vi "Main.vi"(11 "Mode":T1(ring)) -> ()   [LabVIEW 2017]
uses:
  Game Mode/Game Mode.lvclass
  Game Mode/PvP-1/Single Computer PvP.lvclass
  C:/LabVIEW Packages/Sources/GuessingGame/Game Mode/Game Mode.lvclass
panel:
  out "error out":errorcluster
  in  "Stop":bool
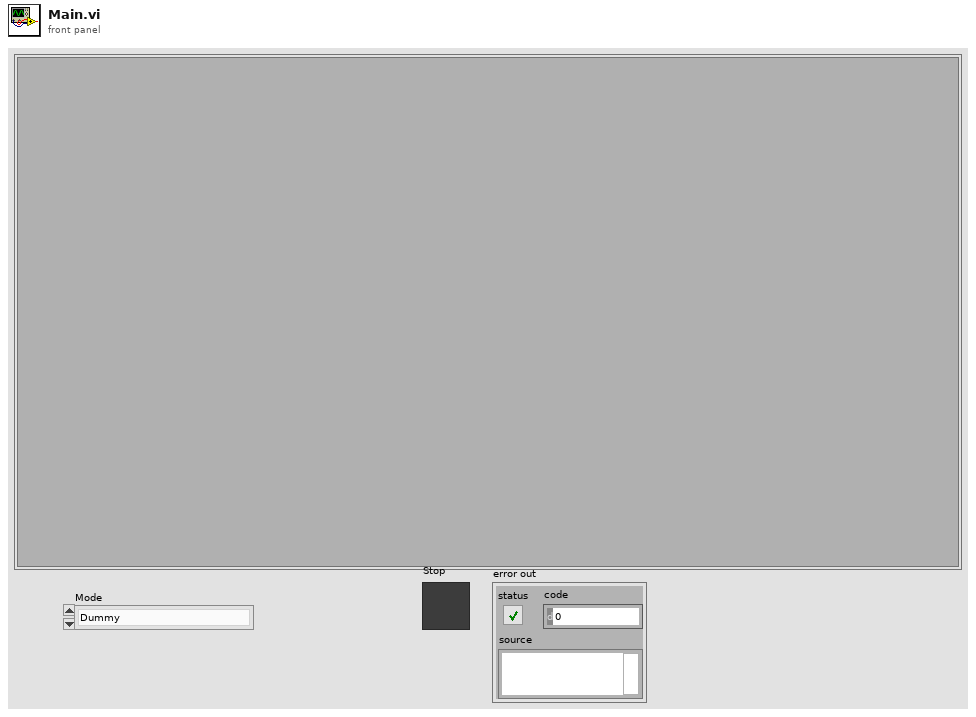
[diagram p1: front panel]
types:
  T1 = enum16{"Dummy", "Single PC - PvP", "Multiple PC - PvP", "Single PC - PvComputer"}
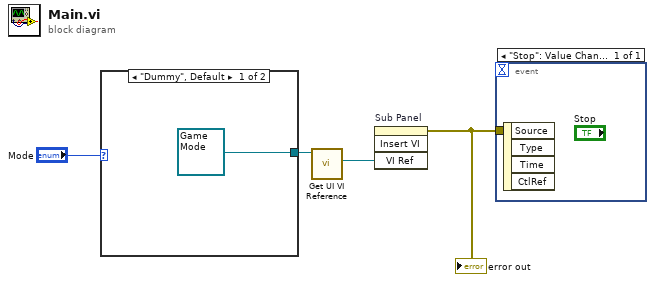
[diagram p0: block diagram]
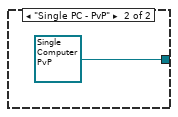
[diagram p2: hidden frame]
diagram:
  n1 = case shown="\"Dummy\", Default" "Mode" {
    tunnel: [refnum<class "Game Mode.lvclass"> refnum ("Game Mode.lvclass") refnum<class "Single Computer PvP.lvclass"> refnum ("Single Computer PvP.lvclass")] -> w3
    frame "Dummy", Default {
    }
    frame "Single PC - PvP" {
    }
  }
  n2 = call-dynamic "Get UI VI Reference.vi"("Game Mode in"=w3) -> ("VI Refnum"=w2:refnum<vi>)  [unwired: 8 in, 2 out]
  n3 = invoke on="Sub Panel" class="SubPnl" method="Insert VI"("VI Ref"=w2) -> (error out=w1:errorcluster)  [unwired: 3 in, 3 out]
  "error out" <- w1
  n4 = event shown="[0] \"Stop\": Value Change" {
    selector: _ -> [_]
    dyn-events: _ -> [_]
    timeout: _ -> [_]
    tunnel: w1 -> [_]
    event "Stop": Value Change {
      n5 = event-data() -> ()  [unwired: 1 in, 4 out]
    }
  }
